vi "captureSpectImage.vi"(8 "error in (no error)":errorcluster, 9 "command_captureSpectImage":T1, 10 "model in":refnum<class "IModel.lvclass">, 11 "NotImagingState in":refnum<class "NotImagingState.lvclass">) -> (0 "error out":errorcluster, 2 "model out":refnum<class "IModel.lvclass">, 3 "NotImagingState out":refnum<class "NotImagingState.lvclass">)   [LabVIEW 2016, in "States.lvlib" / "NotImagingState.lvclass"]
uses:
  NotImagingState.lvclass
  IModel/IModel.lvclass
  ts_sallv_sedspectrometer/DataTypes/command_captureSpectImage.ctl
  Typedefs/CommandValue.ctl
  ts_sallv_sedspectrometer/DataTypes/logevent_DetailedState.ctl
  Typedefs/SEDSpectrometerTypedefs.lvlib
  ts_sallv_sedspectrometer/SALLV_sedSpectrometer.lvlib
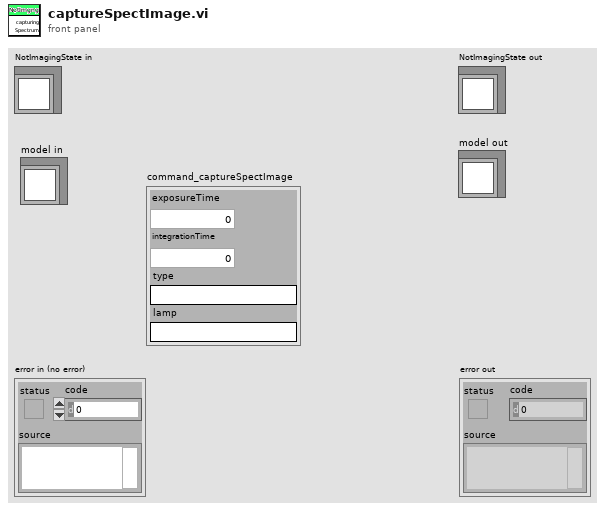
[diagram p1: front panel]
types:
  T1 = typedef "SALLV_sedSpectrometer.lvlib/command_captureSpectImage.ctl" = cluster{"exposureTime":sgl, "integrationTime":sgl, "type":string, "lamp":string}
  T2 = typedef "SALLV_sedSpectrometer.lvlib/logevent_DetailedState.ctl" = cluster{"detailedState":enum32{"", "DisabledState", "EnabledState", "FaultState", "OfflineState", "StandbyState", "CaptureSpectImage", "NotImaging"}, "priority":i32}
  T3 = typedef "SEDSpectrometerTypedefs.lvlib/CommandValue.ctl" = enum16{"clearError", "disable", "enable", "exit", "GoToStandby", "OnHeartbeat", "OnIncomingMessagingError", "OnInterrupt", "start", "captureSpectImage", "setSpectTempSetpoint", "stopImageCapture"}
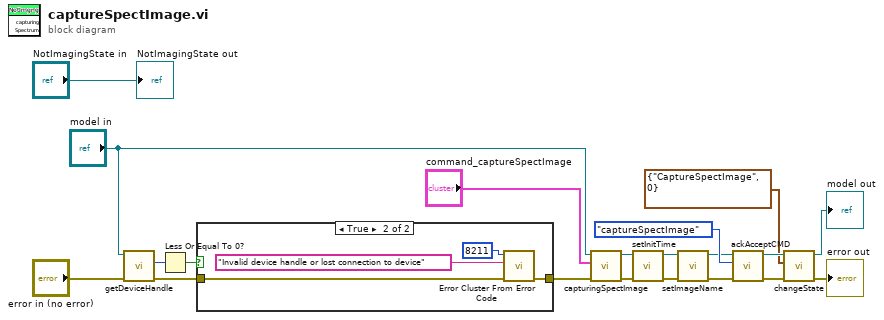
[diagram p0: block diagram]
diagram:
  n1 = call-dynamic "getDeviceHandle.vi"("error in (no error)"="error in (no error)", "IModel in"="model in") -> ("error out"=w13:errorcluster, "Device"=w14:i32)  [unwired: 7 in, 1 out]
  n2 = Less Or Equal To 0?(x=w14) -> (x <= 0?=w12:bool)
  n3 = case shown="True" w12 {
    tunnel: [w21 w23] -> w9
    tunnel: w13 -> [w21 w22]
    frame False {
    }
    frame True {
      n4 = call <vilib>:"Error Cluster From Error Code.vi"("error in (no error)"=w22, "error message (\"\")"="Invalid device handle or lost connection to device" ("error message (\"\")"), "error code (0)"=8211) -> ("error out"=w23:errorcluster)  [unwired: 6 in]
    }
  }
  n5 = call-dynamic "capturingSpectImage.vi"("error in (no error)"=w9, "command_captureSpectImage"="command_captureSpectImage", "IModel in"="model in") -> ("error out"=w7:errorcluster, "IModel out"=w8:refnum<class "IModel.lvclass">)  [unwired: 7 in]
  n6 = call-dynamic "setInitTime.vi"("error in (no error)"=w7, "IModel in"=w8) -> ("error out"=w4:errorcluster, "IModel out"=w5:refnum<class "IModel.lvclass">)  [unwired: 8 in]
  n7 = call-dynamic "setImageName.vi"("error in (no error)"=w4, "IModel in"=w5) -> ("error out"=w1:errorcluster, "IModel out"=w2:refnum<class "IModel.lvclass">)  [unwired: 8 in]
  n8 = call-dynamic "ackAcceptCMD.vi"("error in (no error)"=w1, "CommandValue"=CommandValue."captureSpectImage", "IModel in"=w2) -> ("error out"=w19:errorcluster, "IModel out"=w20:refnum<class "IModel.lvclass">)  [unwired: 7 in]
  n9 = call-dynamic "changeState.vi"("error in (no error)"=w19, "DetailedState"=T2 {"detailedState"=enum."CaptureSpectImage", "priority"=0}, "IModel in"=w20) -> ("error out"=→"error out":errorcluster, "IModel out"=→"model out":refnum<class "IModel.lvclass">)  [unwired: 7 in]
  "NotImagingState out" <- "NotImagingState in"
